vi "FlattenTo1DArray.vi"(11 "Matrix":bool[][](array[boolean])) -> (3 "1D Array":bool[](array[boolean]))   [LabVIEW 2021, in "Bananas.lvlib" / "Pips.lvclass"]
uses:
  Pips.lvclass
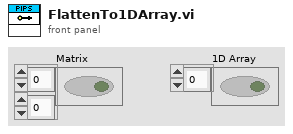
[diagram p1: front panel]
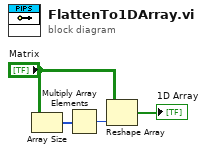
[diagram p0: block diagram]
diagram:
  n1 = Array Size(array="Matrix") -> (size(s)=w1:i32[])
  n2 = Multiply Array Elements(1:w1) -> (0:w2:i32)
  n3 = Reshape Array("Matrix", w2) -> (→"1D Array":bool[])
